vi "Read Enable Server Generic UE.vi"(11 "Template Server in":refnum<class "Template Server.lvclass">) -> (2 "Enable Server Generic UE":bool, 3 "Template Server out":refnum<class "Template Server.lvclass">)   [LabVIEW 2019, in "Template Server.lvlib" / "Template Server.lvclass"]
uses:
  Template Server.lvclass
  Template Server.lvclass/Template Server.ctl
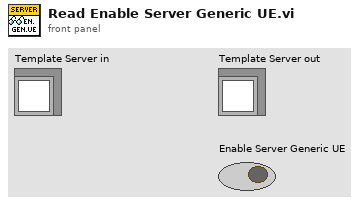
[diagram p1: front panel]
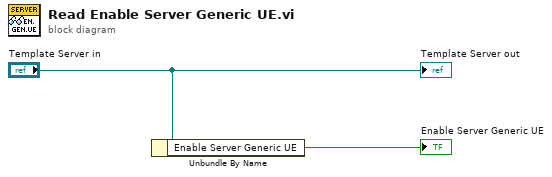
[diagram p0: block diagram]
diagram:
  n1 = Unbundle By Name("Template Server in") -> ("Enable Server Generic UE"=→"Enable Server Generic UE":bool)
  "Template Server out" <- "Template Server in"
